vi "Turn to Angle.vi"(4 "Angle Tolerance":dbl, 5 "PID Gains":T1 {"derivative time (Td, min)" format="%.3f"; "integral time (Ti, min)" format="%.3f"; "proportional gain (Kc)" format="%.3f"}, 6 "Rotation Multiplier":dbl, 7 "Target angle":dbl, 8 "Angle (radians; 0 = right)":dbl) -> (1 "Finished?":bool, 3 "Turn Set Point":dbl)   [LabVIEW 2015]
uses:
  <vilib>/addons/control/pid/pid.llb/PID Control Input Filter (DBL).vi
  <vilib>/addons/control/pid/pid.llb/PID (DBL).vi
  <vilib>/addons/control/pid/NI_PID_pid.lvlib
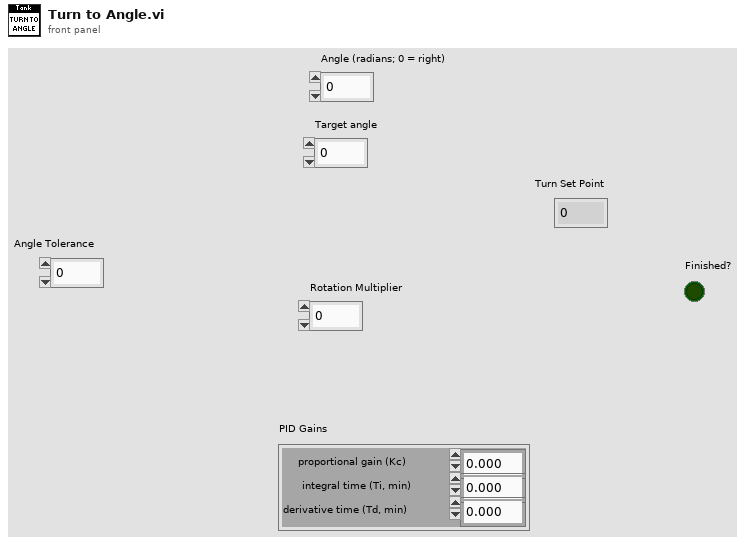
[diagram p1: front panel]
types:
  T1 = cluster{"proportional gain (Kc)":dbl, "integral time (Ti, min)":dbl, "derivative time (Td, min)":dbl}
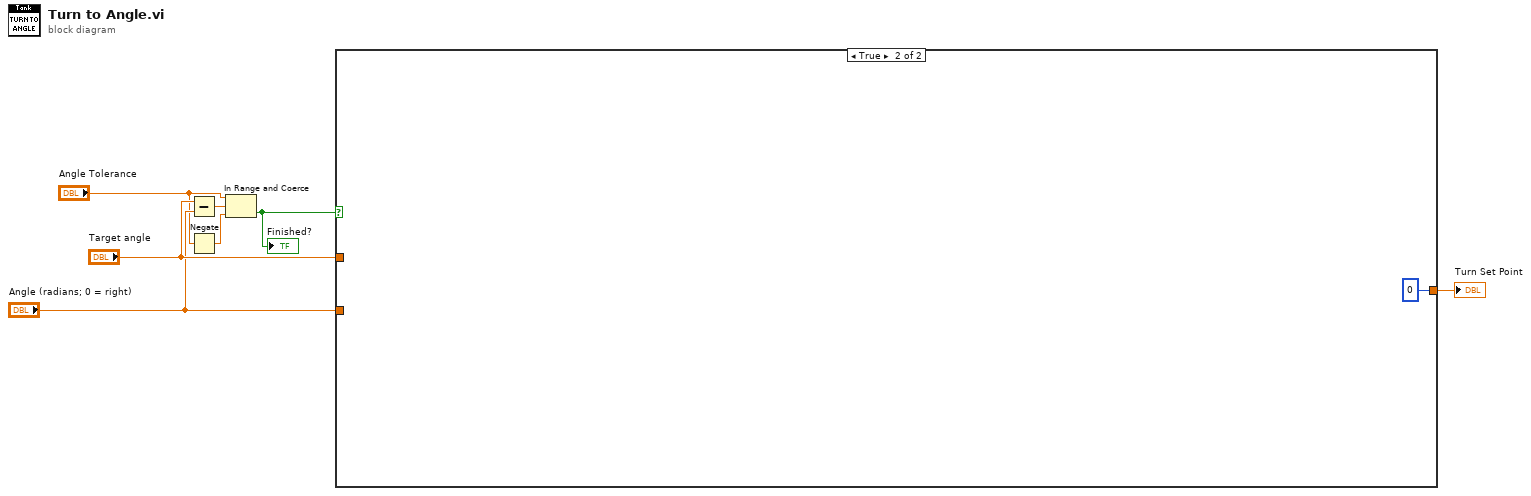
[diagram p0: block diagram]
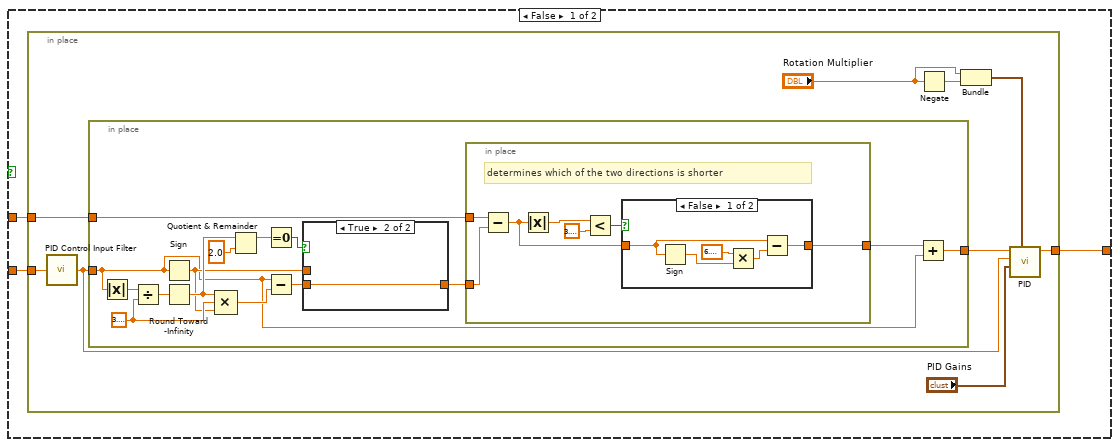
[diagram p2: hidden frame]
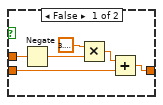
[diagram p4: hidden frame]
diagram:
  n1 = Subtract(x="Target angle", y="Angle (radians; 0 = right)") -> (x-y=w4:dbl)
  n2 = Negate(x="Angle Tolerance") -> (-x=w2:dbl)
  n3 = In Range and Coerce(upper limit="Angle Tolerance", x=w4, lower limit=w2) -> (In Range?=w1:bool)  [unwired: 1 out]
  "Finished?" <- w1
  n4 = case shown="True" w1 {
    tunnel: "Target angle" -> [w10 _]
    tunnel: [w9 0] -> w7
    tunnel: "Angle (radians; 0 = right)" -> [w8 _]
    frame False {
      n5 = in-place {
        in-place-border: [w19] -> w9
        in-place-border: w10 -> [w14]
        in-place-border: w8 -> [w11]
        n6 = call-poly <vilib>:"PID Control Input Filter.vi"("input"=w11) -> ("output"=w12:dbl)  [unwired: 4 in]
        n7 = in-place {
          in-place-border: w14 -> [w23]
          in-place-border: [w22] -> w13
          in-place-border: w12 -> [w20]
          w31 = 3.141592653589793
          n8 = Absolute Value(x=w20) -> (abs(x)=w34:dbl)
          n9 = Divide(x=w34, y=w31) -> (x/y=w33:dbl)
          n10 = Sign(1:w20) -> (0:w25:dbl)
          n11 = Round Toward -Infinity(1:w33) -> (0:w30:dbl)
          n12 = Compound Arithmetic op=MULTIPLY(w30, w31, w25) -> (w32:dbl)
          n13 = Quotient & Remainder(x=w30, y=2.0) -> (x-y*floor(x/y)=w28:dbl)  [unwired: 1 out]
          n14 = Equal To 0?(x=w28) -> (x = 0?=w26:bool)
          n15 = Subtract(x=w20, y=w32) -> (x-y=w27:dbl)
          n16 = case shown="True" w26 {
            tunnel: [w52 w54] -> w24
            tunnel: w27 -> [w53 w54]
            tunnel: w25 -> [w51 _]
            frame False {
              n17 = Negate(x=w51) -> (-x=w49:dbl)
              n18 = Multiply(x=3.141592653589793, y=w49) -> (x*y=w48:dbl)
              n19 = Add(x=w48, y=w53) -> (x+y=w52:dbl)
            }
            frame True {
            }
          }
          n20 = in-place {
            in-place-border: w23 -> [w36]
            in-place-border: w24 -> [w35]
            in-place-border: [w37] -> w21
            # "determines which of the two directions is shorter"
            n21 = Subtract(x=w36, y=w35) -> (x-y=w41:dbl)
            n22 = Absolute Value(x=w41) -> (abs(x)=w40:dbl)
            n23 = Less?(x=w40, y=3.141592653589793) -> (x < y?=w39:bool)
            n24 = case shown="False" w39 {
              tunnel: w41 -> [w43 w47]
              tunnel: [w42 w47] -> w37
              frame False {
                n25 = Sign(1:w43) -> (0:w45:dbl)
                n26 = Multiply(x=6.283185307179586, y=w45) -> (x*y=w44:dbl)
                n27 = Subtract(x=w43, y=w44) -> (x-y=w42:dbl)
              }
              frame True {
              }
            }
          }
          n28 = Add(x=w21, y=w20) -> (x+y=w22:dbl)
        }
        n29 = Negate(x="Rotation Multiplier") -> (-x=w16:dbl)
        n30 = Bundle("Rotation Multiplier"="Rotation Multiplier", w16) -> (w15:cluster{"Rotation Multiplier":dbl, dbl})  [unwired: 1 in]
        n31 = call-poly <vilib>:"PID.vi"("output range"=w15, "PID gains"="PID Gains", "process variable"=w12, "setpoint"=w13) -> ("output"=w19:dbl)  [unwired: 6 in, 1 out]
      }
    }
    frame True {
    }
  }
  "Turn Set Point" <- w7
